vi "GOLPI full test.vi"() -> ()   [LabVIEW 2013]
uses:
  Private/Set Variable - polymorph parts/Set Double.vi
  Private/Get Variable - polymorph parts/Get Double.vi
  Private/Set Variable - polymorph parts/Set Double Complex.vi
  Private/Get Variable - polymorph parts/Get Double Complex.vi
  Private/Set Variable - polymorph parts/Set 2D Array Double.vi
  Private/Get Variable - polymorph parts/Get 2D Array Double.vi
  Private/Set Variable - polymorph parts/Set 2D Array Double Complex.vi
  Private/Get Variable - polymorph parts/Get 2D Array Double Complex.vi
  Private/Set Variable - polymorph parts/Set String.vi
  Private/Get Variable - polymorph parts/Get String.vi
  Private/Set Variable - polymorph parts/Set 1D Array String.vi
  Private/Get Variable - polymorph parts/Get 1D Array String.vi
  GOLPI library.lvlib
panel:
  out "all tests result":bool
  out "test results":T1(array[cluster])
  in  "do tests with large random datasets?":bool
  out "GNU Octave version":string
  out "exit code":i32
  out "error out":errorcluster
  in  "Octave binary directory":path=path "C:/Program Files/Octave-3.6.2/bin"
  in  "Working directory":path=path "C:/"
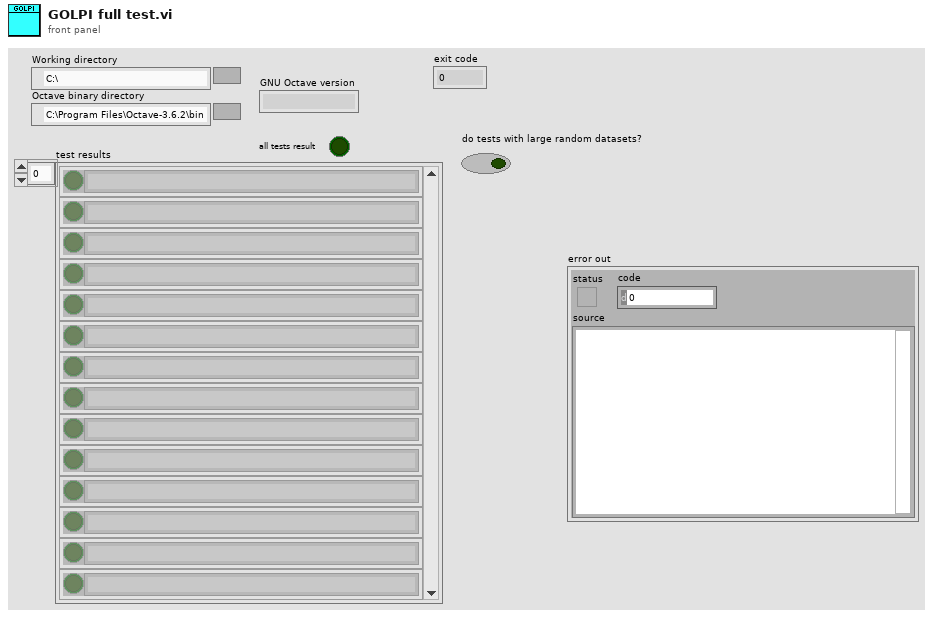
[diagram p1: front panel]
types:
  T1 = cluster{"test result":bool, "variable name":string}[]
  T2 = typedef "GOLPI library.lvlib/GOLPI reference Type Def.ctl" = cluster{"pipe handle":T3, "fast read timeout [ms]":u32, "fast read settle time [ms]":u32, "fast read to multiple [ms]":u32, "max elements per input line":u32}
  T3 = typedef "LV Process.lvlibp/Pipe Handle.ctl" = cluster{"lv_proc.dll file path":path, "process instance handle":u32[]}
  T4 = cluster{"test result":bool, "variable name":string}
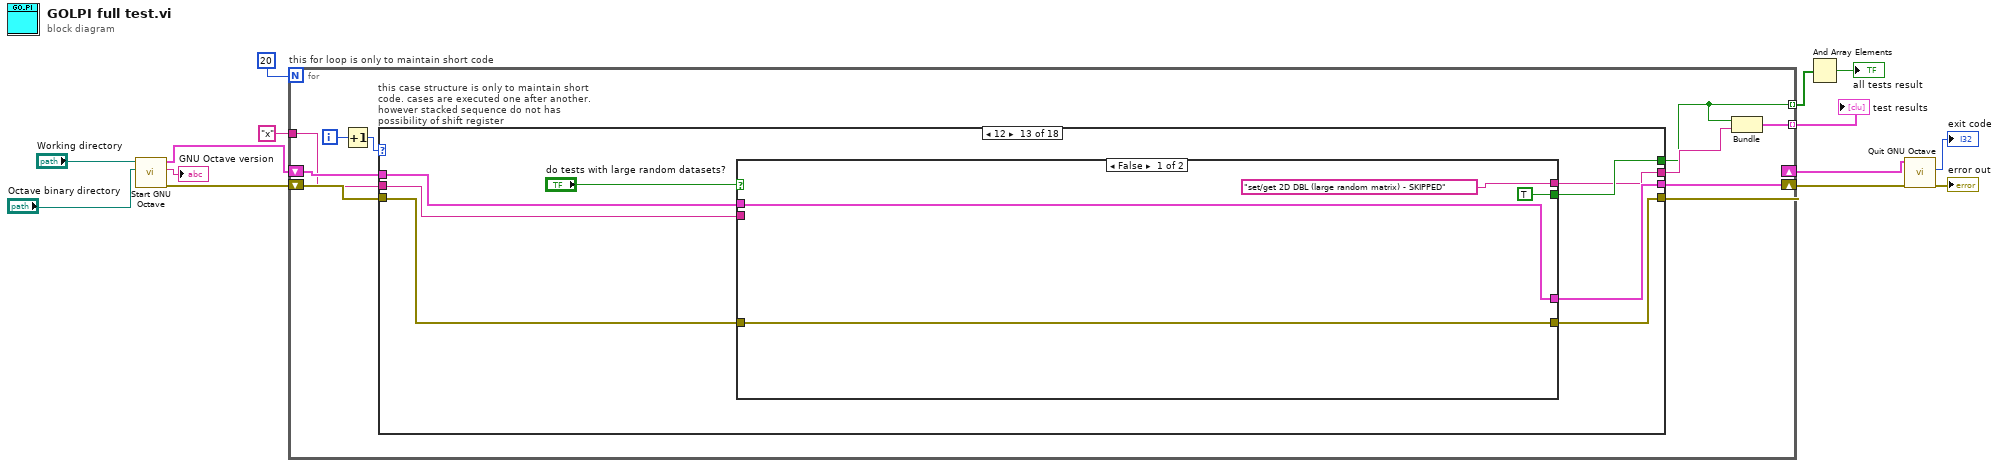
[diagram p0: block diagram]
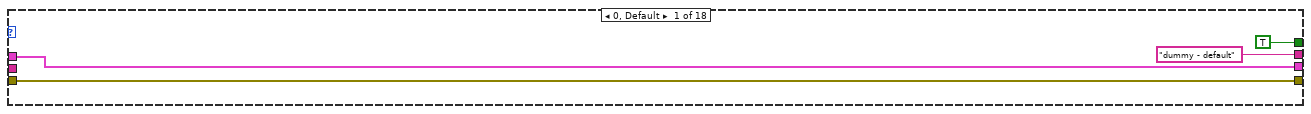
[diagram p2: hidden frame]
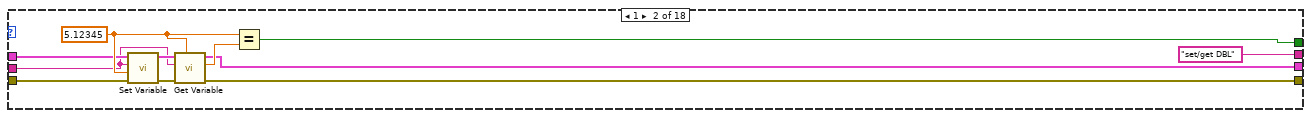
[diagram p3: hidden frame]
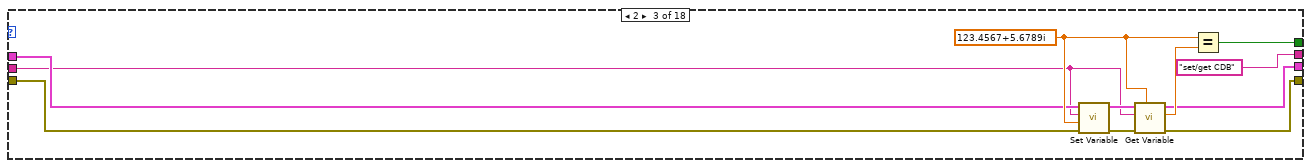
[diagram p4: hidden frame]
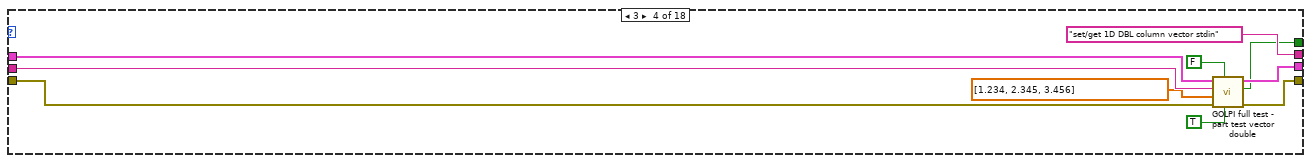
[diagram p5: hidden frame]
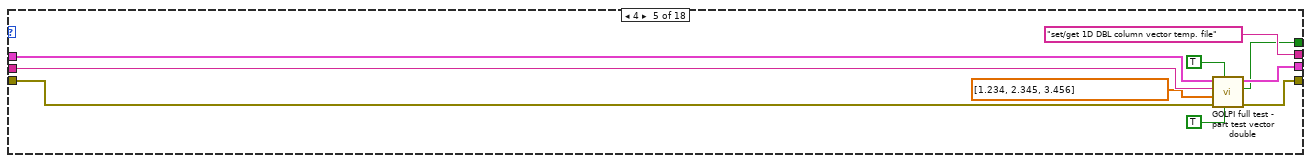
[diagram p6: hidden frame]
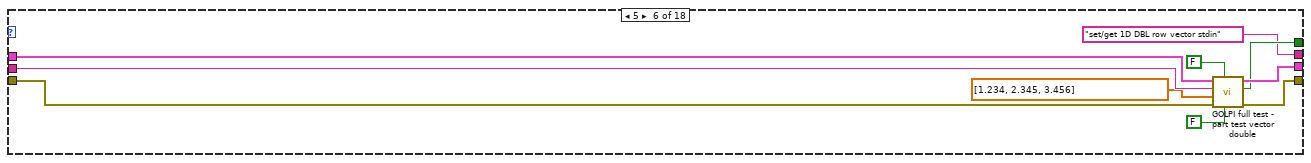
[diagram p7: hidden frame]
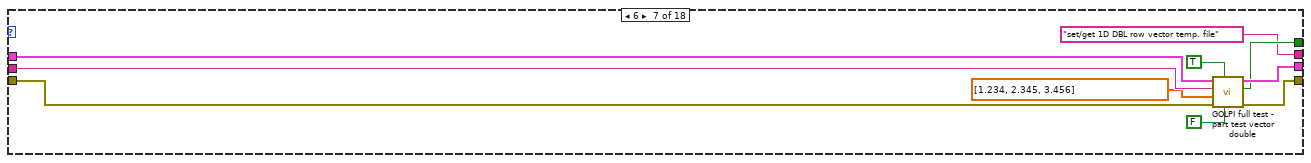
[diagram p8: hidden frame]
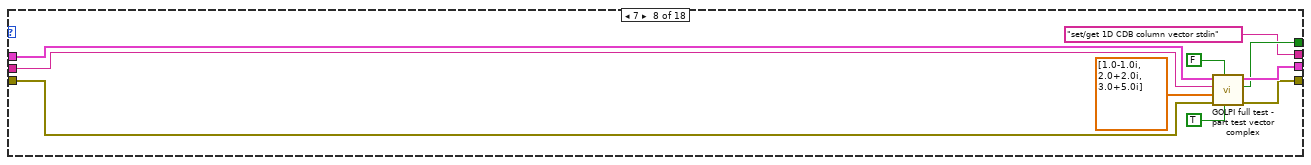
[diagram p9: hidden frame]
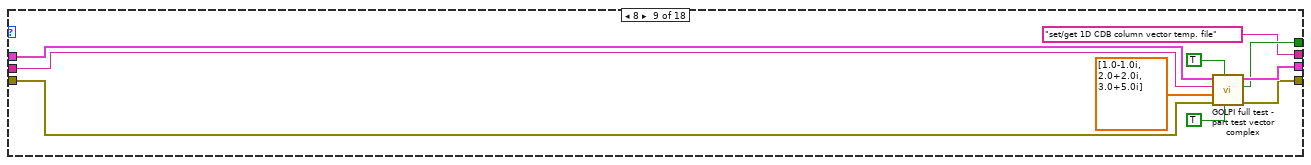
[diagram p10: hidden frame]
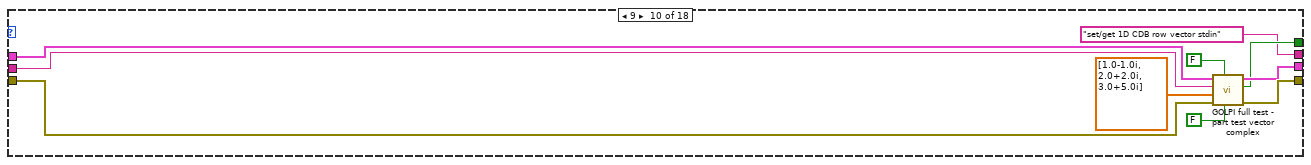
[diagram p11: hidden frame]
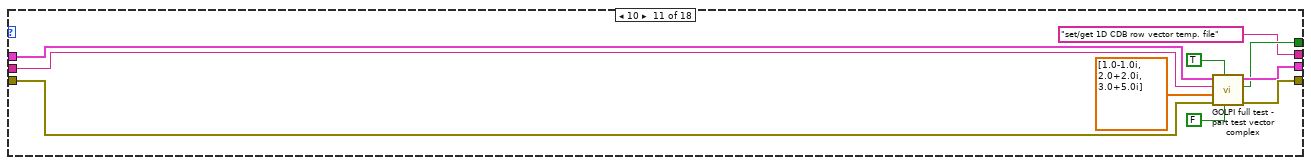
[diagram p12: hidden frame]
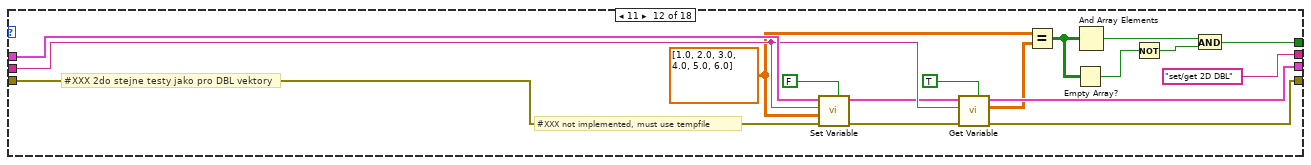
[diagram p13: hidden frame]
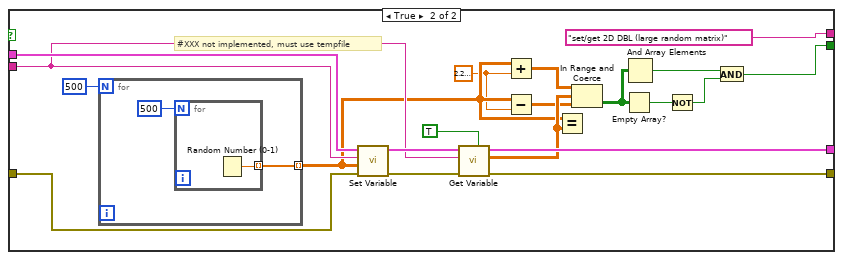
[diagram p14: hidden frame]
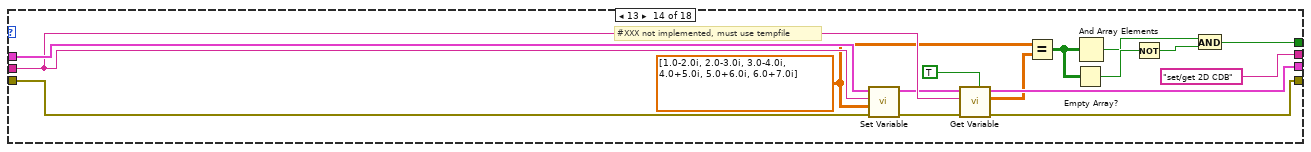
[diagram p15: hidden frame]
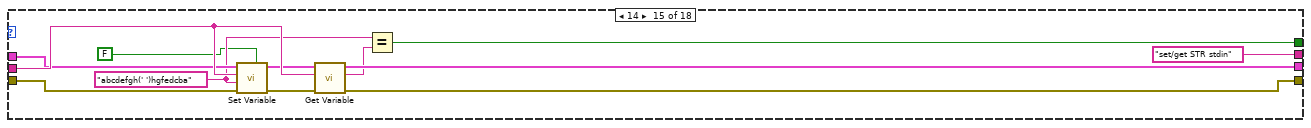
[diagram p16: hidden frame]
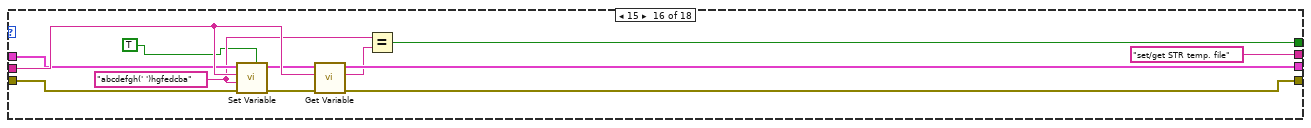
[diagram p17: hidden frame]
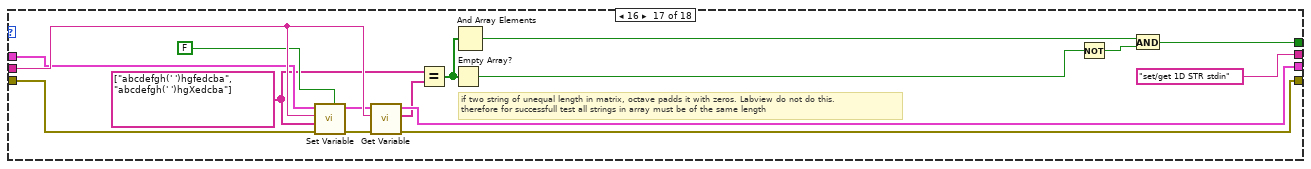
[diagram p18: hidden frame]
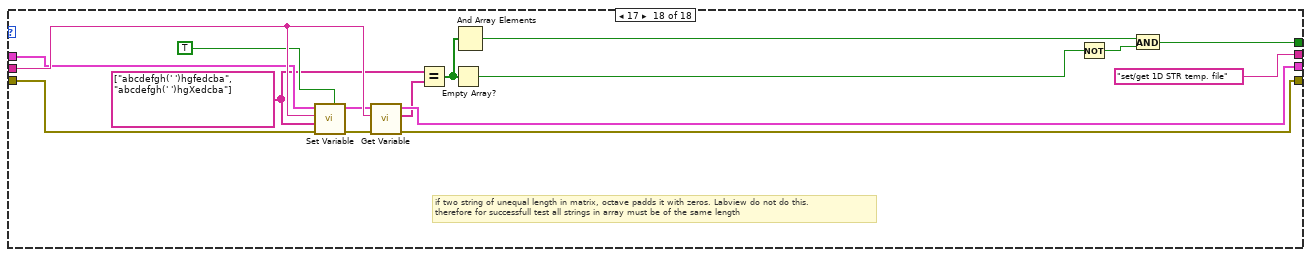
[diagram p19: hidden frame]
diagram:
  n1 = call "Start GNU Octave.vi"("Octave binary directory"="Octave binary directory", "Working directory"="Working directory") -> ("error out"=w8:errorcluster, "GNU Octave version"=→"GNU Octave version":string, "GOLPI ref. out"=w9:T2)  [unwired: 6 in, 1 out]
  n2 = for "this for loop is only to maintain short code" {
    N: 20 -> [_]
    tunnel: "x" ("variable name") -> [w22]
    shift-right: [w21] -> w5
    shift-left: w8 -> [w23]
    shift-right: [w20] -> w6
    shift-left: w9 -> [w24]
    tunnel: [w16] -> w3 mode=indexing
    tunnel: [w15] -> w2 mode=indexing
    i -> [w19]
    n3 = Increment(x=w19) -> (x+1=w18:i32)
    n4 = case "this case structure is only to maintain short code. cases are executed one after another. however stacked sequence do not has possibility of shift register" shown="12" w18 {
      tunnel: w24 -> [w27 w35 w42 w56 w66 w78 w88 w99 w109 w117 w127 w143 w151 w197 w207 w219 w235 w251]
      tunnel: w23 -> [w28 w34 w43 w59 w69 w80 w90 w96 w106 w120 w130 w144 w152 w198 w208 w220 w236 w252]
      tunnel: [w28 w33 w44 w58 w68 w77 w87 w97 w107 w119 w129 w146 w154 w196 w205 w217 w233 w249] -> w21
      tunnel: [w27 w32 w45 w57 w67 w75 w85 w98 w108 w118 w128 w145 w153 w195 w204 w216 w232 w248] -> w20
      tunnel: w22 -> [_ w31 w41 w55 w65 w79 w89 w95 w105 w116 w126 w142 w150 w194 w209 w221 w237 w253]
      tunnel: [TRUE w30 w46 w51 w61 w74 w84 w93 w103 w112 w122 w147 w155 w193 w199 w212 w223 w239] -> w15
      tunnel: ["dummy - default" ("variable name") "set/get DBL" ("variable name") "set/get CDB" ("variable name") "set/get 1D DBL column vector stdin" ("variable name") "set/get 1D DBL column vector temp. file" ("variable name") "set/get 1D DBL row vector stdin" ("variable name") "set/get 1D DBL row vector temp. file" ("variable name") "set/get 1D CDB column vector stdin" ("variable name") "set/get 1D CDB column vector temp. file" ("variable name") "set/get 1D CDB row vector stdin" ("variable name") "set/get 1D CDB row vector temp. file" ("variable name") "set/get 2D DBL" ("variable name") w149 "set/get 2D CDB" ("variable name") "set/get STR stdin" ("variable name") "set/get STR temp. file" ("variable name") "set/get 1D STR stdin" ("variable name") "set/get 1D STR temp. file" ("variable name")] -> w17
      frame 0, Default {
      }
      frame 1 {
        w36 = 5.12345 ("value")
        n5 = call-poly "Set Variable.vi"("error in"=w34, "value"=w36, "variable name"=w31, "GOLPI ref. in"=w35) -> ("error out"=w38:errorcluster, "GOLPI ref. out"=w39:T2)  [unwired: 6 in]
        n6 = call-poly "Get Variable.vi"("data type of variable"=w36, "error in"=w38, "variable name"=w31, "GOLPI ref. in"=w39) -> ("error out"=w33:errorcluster, "value"=w37:dbl, "GOLPI ref. out"=w32:T2)  [unwired: 5 in]
        n7 = Equal?(x=w36, y=w37) -> (x = y?=w30:bool)
      }
      frame 2 {
        w49 = cdb 123.4567+5.6789i ("value")
        n8 = call-poly "Set Variable.vi"("error in"=w43, "value"=w49, "variable name"=w41, "GOLPI ref. in"=w42) -> ("error out"=w48:errorcluster, "GOLPI ref. out"=w47:T2)  [unwired: 6 in]
        n9 = call-poly "Get Variable.vi"("data type of variable"=w49, "error in"=w48, "variable name"=w41, "GOLPI ref. in"=w47) -> ("error out"=w44:errorcluster, "value"=w50:cdb, "GOLPI ref. out"=w45:T2)  [unwired: 5 in]
        n10 = Equal?(x=w49, y=w50) -> (x = y?=w46:bool)
      }
      frame 3 {
        n11 = call "GOLPI full test - part test vector double.vi"("column vector?"=TRUE, "set: use temporary file?"=FALSE, "error in (no error)"=w59, "test value"=dbl[] [1.234, 2.345, 3.456] ("value"), "variable name in"=w55, "GOLPI ref. in"=w56) -> ("error out"=w58:errorcluster, "test result"=w51:bool, "GOLPI ref. out"=w57:T2)  [unwired: 3 in]
      }
      frame 4 {
        n12 = call "GOLPI full test - part test vector double.vi"("column vector?"=TRUE, "set: use temporary file?"=TRUE, "error in (no error)"=w69, "test value"=dbl[] [1.234, 2.345, 3.456] ("value"), "variable name in"=w65, "GOLPI ref. in"=w66) -> ("error out"=w68:errorcluster, "test result"=w61:bool, "GOLPI ref. out"=w67:T2)  [unwired: 3 in]
      }
      frame 5 {
        n13 = call "GOLPI full test - part test vector double.vi"("column vector?"=FALSE, "set: use temporary file?"=FALSE, "error in (no error)"=w80, "test value"=dbl[] [1.234, 2.345, 3.456] ("value"), "variable name in"=w79, "GOLPI ref. in"=w78) -> ("error out"=w77:errorcluster, "test result"=w74:bool, "GOLPI ref. out"=w75:T2)  [unwired: 3 in]
      }
      frame 6 {
        n14 = call "GOLPI full test - part test vector double.vi"("column vector?"=FALSE, "set: use temporary file?"=TRUE, "error in (no error)"=w90, "test value"=dbl[] [1.234, 2.345, 3.456] ("value"), "variable name in"=w89, "GOLPI ref. in"=w88) -> ("error out"=w87:errorcluster, "test result"=w84:bool, "GOLPI ref. out"=w85:T2)  [unwired: 3 in]
      }
      frame 7 {
        n15 = call "GOLPI full test - part test vector complex.vi"("column vector?"=TRUE, "set: use temporary file?"=FALSE, "error in (no error)"=w96, "test value"=cdb[] [1.0-1.0i, 2.0+2.0i, 3.0+5.0i] ("value"), "variable name in"=w95, "GOLPI ref. in"=w99) -> ("error out"=w97:errorcluster, "test result"=w93:bool, "GOLPI ref. out"=w98:T2)  [unwired: 3 in]
      }
      frame 8 {
        n16 = call "GOLPI full test - part test vector complex.vi"("column vector?"=TRUE, "set: use temporary file?"=TRUE, "error in (no error)"=w106, "test value"=cdb[] [1.0-1.0i, 2.0+2.0i, 3.0+5.0i] ("value"), "variable name in"=w105, "GOLPI ref. in"=w109) -> ("error out"=w107:errorcluster, "test result"=w103:bool, "GOLPI ref. out"=w108:T2)  [unwired: 3 in]
      }
      frame 9 {
        n17 = call "GOLPI full test - part test vector complex.vi"("column vector?"=FALSE, "set: use temporary file?"=FALSE, "error in (no error)"=w120, "test value"=cdb[] [1.0-1.0i, 2.0+2.0i, 3.0+5.0i] ("value"), "variable name in"=w116, "GOLPI ref. in"=w117) -> ("error out"=w119:errorcluster, "test result"=w112:bool, "GOLPI ref. out"=w118:T2)  [unwired: 3 in]
      }
      frame 10 {
        n18 = call "GOLPI full test - part test vector complex.vi"("column vector?"=FALSE, "set: use temporary file?"=TRUE, "error in (no error)"=w130, "test value"=cdb[] [1.0-1.0i, 2.0+2.0i, 3.0+5.0i] ("value"), "variable name in"=w126, "GOLPI ref. in"=w127) -> ("error out"=w129:errorcluster, "test result"=w122:bool, "GOLPI ref. out"=w128:T2)  [unwired: 3 in]
      }
      frame 11 {
        w134 = dbl[][] [[1.0, 2.0, 3.0], [4.0, 5.0, 6.0]] ("value")
        # "#XXX 2do stejne testy jako pro DBL vektory"
        # "#XXX not implemented, must use tempfile"
        n19 = call-poly "Set Variable.vi"("use temporary file?"=FALSE, "error in"=w144, "value"=w134, "variable name"=w142, "GOLPI ref. in"=w143) -> ("error out"=w132:errorcluster, "GOLPI ref. out"=w131:T2)  [unwired: 5 in]
        n20 = call-poly "Get Variable.vi"("use temporary file?"=TRUE, "error in"=w132, "variable name"=w142, "GOLPI ref. in"=w131) -> ("error out"=w146:errorcluster, "value"=w135:dbl[][], "GOLPI ref. out"=w145:T2)  [unwired: 5 in]
        n21 = Equal?(x=w134, y=w135) -> (x = y?=w137:bool[][])
        n22 = Empty Array?(array=w137) -> (empty?=w138:bool)
        n23 = And Array Elements(Boolean array=w137) -> (logical AND=w140:bool)
        n24 = Not(x=w138) -> (.not. x?=w139:bool)
        n25 = And(x=w140, y=w139) -> (x .and. y?=w147:bool)
      }
      frame 12 {
        n26 = case shown="False" "do tests with large random datasets?" {
          tunnel: [TRUE w173] -> w155
          tunnel: [w159 w172] -> w154
          tunnel: [w158 w171] -> w153
          tunnel: w152 -> [w159 w170]
          tunnel: w151 -> [w158 w169]
          tunnel: w150 -> [_ w168]
          tunnel: ["set/get 2D DBL (large random matrix) - SKIPPED" ("variable name") "set/get 2D DBL (large random matrix)" ("variable name")] -> w149
          frame False {
          }
          frame True {
            w162 = 2.220446049250313e-16
            # "#XXX not implemented, must use tempfile"
            n27 = for {
              N: 500 ("dimension size") -> [_]
              tunnel: [w181] -> w163 mode=indexing
              n28 = for {
                N: 500 ("dimension size") -> [_]
                tunnel: [w182] -> w181 mode=indexing
                n29 = Random Number (0-1)() -> (number: 0 to 1=w182:dbl)
              }
            }
            n30 = call-poly "Set Variable.vi"("error in"=w170, "value"=w163, "variable name"=w168, "GOLPI ref. in"=w169) -> ("error out"=w174:errorcluster, "GOLPI ref. out"=w175:T2)  [unwired: 6 in]
            n31 = call-poly "Get Variable.vi"("use temporary file?"=TRUE, "error in"=w174, "variable name"=w168, "GOLPI ref. in"=w175) -> ("error out"=w172:errorcluster, "value"=w164:dbl[][], "GOLPI ref. out"=w171:T2)  [unwired: 5 in]
            n32 = Add(x=w163, y=w162) -> (x+y=w165:dbl[][])
            n33 = Subtract(x=w163, y=w162) -> (x-y=w161:dbl[][])
            n34 = Equal?(x=w163, y=w164) -> ()  [unwired: 1 out]
            n35 = In Range and Coerce(upper limit=w165, x=w164, lower limit=w161) -> (In Range?=w160:bool[][])  [unwired: 1 out]
            n36 = Empty Array?(array=w160) -> (empty?=w177:bool)
            n37 = And Array Elements(Boolean array=w160) -> (logical AND=w179:bool)
            n38 = Not(x=w177) -> (.not. x?=w178:bool)
            n39 = And(x=w179, y=w178) -> (x .and. y?=w173:bool)
          }
        }
      }
      frame 13 {
        w189 = cdb[][] [[1.0-2.0i, 2.0-3.0i, 3.0-4.0i], [4.0+5.0i, 5.0+6.0i, 6.0+7.0i]] ("value")
        # "#XXX not implemented, must use tempfile"
        n40 = call-poly "Set Variable.vi"("error in"=w198, "value"=w189, "variable name"=w194, "GOLPI ref. in"=w197) -> ("error out"=w191:errorcluster, "GOLPI ref. out"=w190:T2)  [unwired: 6 in]
        n41 = call-poly "Get Variable.vi"("use temporary file?"=TRUE, "error in"=w191, "variable name"=w194, "GOLPI ref. in"=w190) -> ("error out"=w196:errorcluster, "value"=w188:cdb[][], "GOLPI ref. out"=w195:T2)  [unwired: 5 in]
        n42 = Equal?(x=w189, y=w188) -> (x = y?=w186:bool[][])
        n43 = Empty Array?(array=w186) -> (empty?=w185:bool)
        n44 = And Array Elements(Boolean array=w186) -> (logical AND=w183:bool)
        n45 = Not(x=w185) -> (.not. x?=w184:bool)
        n46 = And(x=w183, y=w184) -> (x .and. y?=w193:bool)
      }
      frame 14 {
        w201 = "abcdefgh(' ')hgfedcba" ("value")
        n47 = call-poly "Set Variable.vi"("use temporary file?"=FALSE, "error in"=w208, "value"=w201, "variable name"=w209, "GOLPI ref. in"=w207) -> ("error out"=w210:errorcluster, "GOLPI ref. out"=w206:T2)  [unwired: 5 in]
        n48 = call-poly "Get Variable.vi"("error in"=w210, "variable name"=w209, "GOLPI ref. in"=w206) -> ("error out"=w205:errorcluster, "value"=w203:string, "GOLPI ref. out"=w204:T2)  [unwired: 6 in]
        n49 = Equal?(x=w201, y=w203) -> (x = y?=w199:bool)
      }
      frame 15 {
        w213 = "abcdefgh(' ')hgfedcba" ("value")
        n50 = call-poly "Set Variable.vi"("use temporary file?"=TRUE, "error in"=w220, "value"=w213, "variable name"=w221, "GOLPI ref. in"=w219) -> ("error out"=w222:errorcluster, "GOLPI ref. out"=w218:T2)  [unwired: 5 in]
        n51 = call-poly "Get Variable.vi"("error in"=w222, "variable name"=w221, "GOLPI ref. in"=w218) -> ("error out"=w217:errorcluster, "value"=w215:string, "GOLPI ref. out"=w216:T2)  [unwired: 6 in]
        n52 = Equal?(x=w213, y=w215) -> (x = y?=w212:bool)
      }
      frame 16 {
        w228 = string[] ["abcdefgh(' ')hgfedcba", "abcdefgh(' ')hgXedcba"]
        # "if two string of unequal length in matrix, octave padds it with zeros. Labview do not do this.\ntherefore for successfull test all strings in array must be of the same length"
        n53 = call-poly "Set Variable.vi"("use temporary file?"=FALSE ("use temporary file? 2"), "error in"=w236, "value"=w228, "variable name"=w237, "GOLPI ref. in"=w235) -> ("error out"=w238:errorcluster, "GOLPI ref. out"=w234:T2)  [unwired: 5 in]
        n54 = call-poly "Get Variable.vi"("error in"=w238, "variable name"=w237, "GOLPI ref. in"=w234) -> ("error out"=w233:errorcluster, "value"=w231:string[], "GOLPI ref. out"=w232:T2)  [unwired: 6 in]
        n55 = Equal?(x=w228, y=w231) -> (x = y?=w224:bool[])
        n56 = Empty Array?(array=w224) -> (empty?=w225:bool)
        n57 = And Array Elements(Boolean array=w224) -> (logical AND=w227:bool)
        n58 = Not(x=w225) -> (.not. x?=w226:bool)
        n59 = And(x=w227, y=w226) -> (x .and. y?=w223:bool)
      }
      frame 17 {
        w244 = string[] ["abcdefgh(' ')hgfedcba", "abcdefgh(' ')hgXedcba"]
        # "if two string of unequal length in matrix, octave padds it with zeros. Labview do not do this.\ntherefore for successfull test all strings in array must be of the same length"
        n60 = call-poly "Set Variable.vi"("use temporary file?"=TRUE ("use temporary file? 2"), "error in"=w252, "value"=w244, "variable name"=w253, "GOLPI ref. in"=w251) -> ("error out"=w254:errorcluster, "GOLPI ref. out"=w250:T2)  [unwired: 5 in]
        n61 = call-poly "Get Variable.vi"("error in"=w254, "variable name"=w253, "GOLPI ref. in"=w250) -> ("error out"=w249:errorcluster, "value"=w247:string[], "GOLPI ref. out"=w248:T2)  [unwired: 6 in]
        n62 = Equal?(x=w244, y=w247) -> (x = y?=w240:bool[])
        n63 = Empty Array?(array=w240) -> (empty?=w241:bool)
        n64 = And Array Elements(Boolean array=w240) -> (logical AND=w243:bool)
        n65 = Not(x=w241) -> (.not. x?=w242:bool)
        n66 = And(x=w243, y=w242) -> (x .and. y?=w239:bool)
      }
    }
    n67 = Bundle("test result"=w15, "variable name"=w17) -> (w16:T4)  [unwired: 1 in]
  }
  "test results" <- w3
  n68 = And Array Elements(Boolean array=w2) -> (logical AND=→"all tests result":bool)
  n69 = call "Quit GNU Octave.vi"("error in"=w5, "GOLPI ref. in"=w6) -> ("error out"=→"error out":errorcluster, "exit code"=→"exit code":i32)  [unwired: 8 in]
